vi "CHD_DRIVE_DASH_WRITE.vi"   [LabVIEW 2019]
uses:
  CHD_DRIVE_GLOBALS.vi
  <vilib>/Rock Robotics/Network Tables/NT Write Numeric Array.vi
  <vilib>/Rock Robotics/Network Tables/NT Write Number.vi
  <vilib>/Rock Robotics/WPI/ThirdParty/JAS_Junk/TrajLib/Trajectory_Library.lvlib
types:
  T1 = typedef "Trajectory_Library.lvlib/CHASSIS_SPEEDS.ctl" = cluster{"vX":dbl, "vY":dbl, "vOmega":dbl}
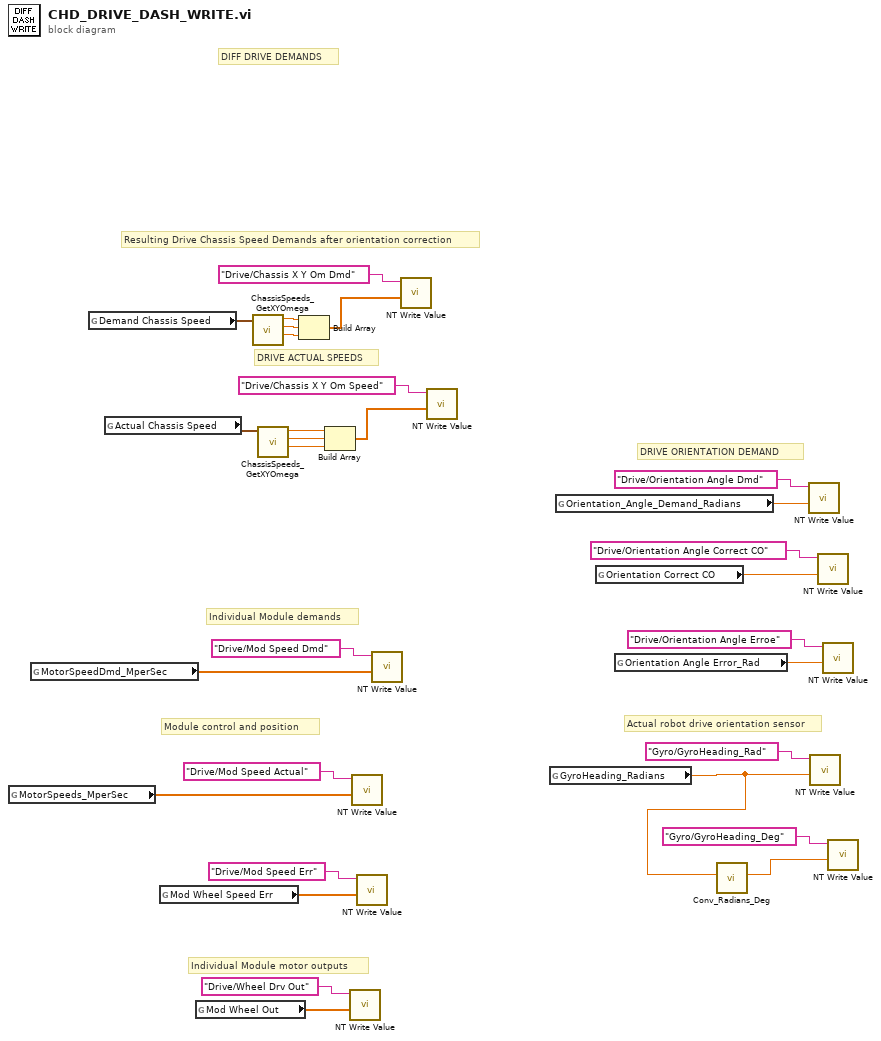
[diagram p0: block diagram]
diagram:
  # "Module control and position"
  # "Actual robot drive orientation sensor"
  # "DRIVE ACTUAL SPEEDS"
  # "DRIVE ORIENTATION DEMAND"
  # "Individual Module motor outputs"
  # "Individual Module demands"
  # "Resulting Drive Chassis Speed Demands after orientation correction"
  # "DIFF DRIVE DEMANDS"
  n1 = global read "CHD_DRIVE_GLOBALS.vi" "MotorSpeeds_MperSec"() -> (w2:dbl[])
  n2 = global read "CHD_DRIVE_GLOBALS.vi" "MotorSpeedDmd_MperSec"() -> (w1:dbl[])
  n3 = global read "CHD_DRIVE_GLOBALS.vi" "Demand Chassis Speed"() -> (w10:T1)
  n4 = global read "CHD_DRIVE_GLOBALS.vi" "Actual Chassis Speed"() -> (w6:T1)
  n5 = global read "CHD_DRIVE_GLOBALS.vi" "Mod Wheel Speed Err"() -> (w18:dbl[])
  n6 = global read "CHD_DRIVE_GLOBALS.vi" "Mod Wheel Out"() -> (w17:dbl[])
  n7 = call <vilib>:"ChassisSpeeds_GetXYOmega.vi"("CHASSIS"=w10) -> ("vAngular"=w7:dbl, "vY"=w8:dbl, "vX"=w9:dbl)  [unwired: 8 in]
  n8 = call <vilib>:"ChassisSpeeds_GetXYOmega.vi"("CHASSIS"=w6) -> ("vAngular"=w3:dbl, "vY"=w4:dbl, "vX"=w5:dbl)  [unwired: 8 in]
  n9 = Build Array(w9, w8, w7) -> (w22:dbl[])
  n10 = Build Array(w5, w4, w3) -> (w27:dbl[])
  n11 = call-poly <vilib>:"NT Write Value.vi"("value"=w17, "name"="Drive/Wheel Drv Out" ("Name")) -> ()  [unwired: 9 in, 1 out]
  n12 = call-poly <vilib>:"NT Write Value.vi"("value"=w2, "name"="Drive/Mod Speed Actual" ("Name")) -> ()  [unwired: 9 in, 1 out]
  n13 = call-poly <vilib>:"NT Write Value.vi"("value"=w18, "name"="Drive/Mod Speed Err" ("Name")) -> ()  [unwired: 9 in, 1 out]
  n14 = call-poly <vilib>:"NT Write Value.vi"("value"=w1, "name"="Drive/Mod Speed Dmd" ("Name")) -> ()  [unwired: 9 in, 1 out]
  n15 = call-poly <vilib>:"NT Write Value.vi"("value"=w22, "name"="Drive/Chassis X Y Om Dmd" ("Name")) -> ()  [unwired: 9 in, 1 out]
  n16 = call-poly <vilib>:"NT Write Value.vi"("value"=w27, "name"="Drive/Chassis X Y Om Speed" ("Name")) -> ()  [unwired: 9 in, 1 out]
  n17 = global read "CHD_DRIVE_GLOBALS.vi" "GyroHeading_Radians"() -> (w11:dbl)
  n18 = global read "CHD_DRIVE_GLOBALS.vi" "Orientation_Angle_Demand_Radians"() -> (w16:dbl)
  n19 = global read "CHD_DRIVE_GLOBALS.vi" "Orientation Correct CO"() -> (w15:dbl)
  n20 = global read "CHD_DRIVE_GLOBALS.vi" "Orientation Angle Error_Rad"() -> (w14:dbl)
  n21 = call <vilib>:"Conv_Radians_Deg.vi"("Radians"=w11) -> ("Degrees"=w12:dbl)  [unwired: 10 in]
  n22 = call-poly <vilib>:"NT Write Value.vi"("value"=w16, "name"="Drive/Orientation Angle Dmd" ("Name")) -> ()  [unwired: 9 in, 1 out]
  n23 = call-poly <vilib>:"NT Write Value.vi"("value"=w11, "name"="Gyro/GyroHeading_Rad" ("Name")) -> ()  [unwired: 9 in, 1 out]
  n24 = call-poly <vilib>:"NT Write Value.vi"("value"=w15, "name"="Drive/Orientation Angle Correct CO" ("Name")) -> ()  [unwired: 9 in, 1 out]
  n25 = call-poly <vilib>:"NT Write Value.vi"("value"=w14, "name"="Drive/Orientation Angle Erroe" ("Name")) -> ()  [unwired: 9 in, 1 out]
  n26 = call-poly <vilib>:"NT Write Value.vi"("value"=w12, "name"="Gyro/GyroHeading_Deg" ("Name")) -> ()  [unwired: 9 in, 1 out]
